vi "ReadDB.vi"() -> ()   [LabVIEW 2018]
uses:
  <vilib>/addons/database/Connection.llb/DB Tools Open Connec (Path).vi
  <vilib>/addons/database/_DB Variant To Data/Database Variant To Data.xnode
  <vilib>/addons/database/NI_Database_API.lvlib
panel:
  out "条目数":i32
  out "data":T1(array[cluster])
  out "error out":errorcluster
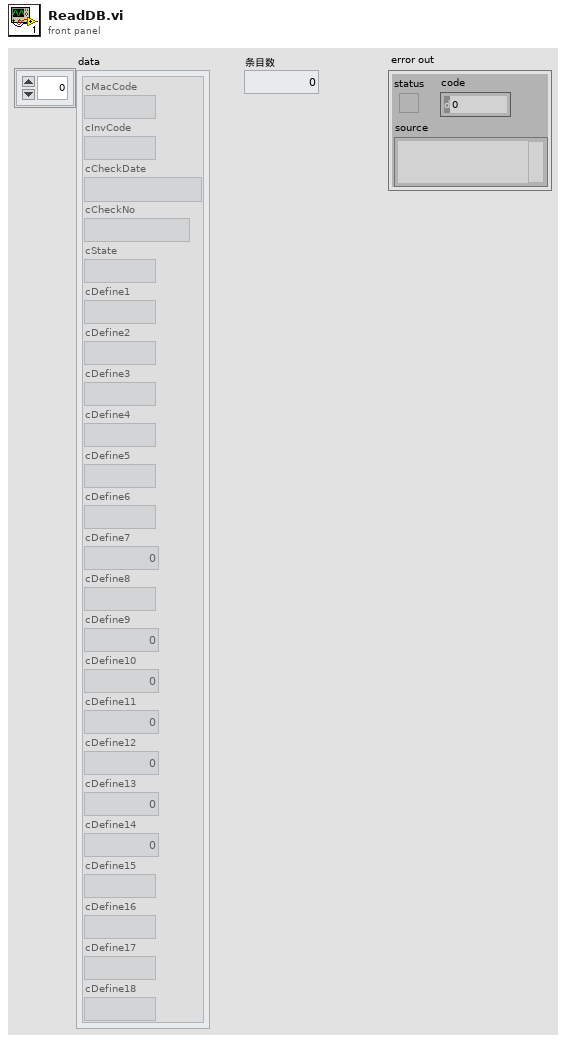
[diagram p1: front panel]
types:
  T1 = cluster{"cMacCode":string, "cInvCode":string, "cCheckDate":string, "cCheckNo":string, "cState":string, "cDefine1":string, "cDefine2":string, "cDefine3":string, "cDefine4":string, "cDefine5":string, "cDefine6":string, "cDefine7":dbl, "cDefine8":string, "cDefine9":dbl, "cDefine10":dbl, "cDefine11":dbl, "cDefine12":dbl, "cDefine13":dbl, "cDefine14":dbl, "cDefine15":string, "cDefine16":string, "cDefine17":string, "cDefine18":string}[]
  T2 = typedef "NI_Database_API.lvlib/Conn ObjectReference.ctl" = refnum<k1>
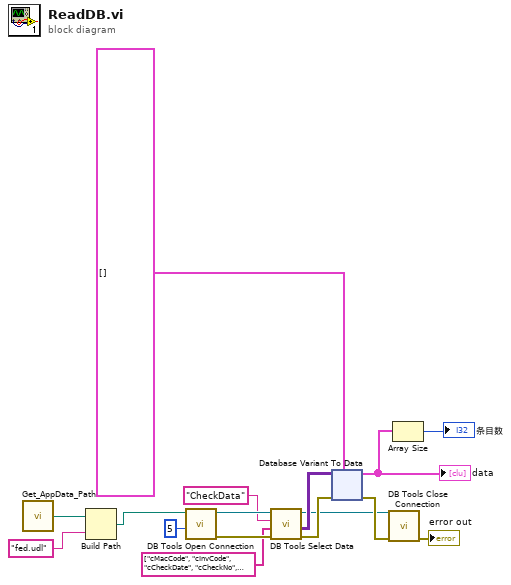
[diagram p0: block diagram]
diagram:
  n1 = call "Get_AppData_Path.vi"() -> ("path"=w15:path)  [unwired: 1 in]
  n2 = Build Path(base path=w15, name or relative path="fed.udl" ("名称或相对路径")) -> (appended path=w14:path)
  n3 = call-poly <vilib>:"DB Tools Open Connection.vi"("connection timeout (15)"=5, "connection information"=w14) -> ("error out"=w10:errorcluster, "connection reference"=w11:T2)  [unwired: 6 in]
  n4 = call <vilib>:"DB Tools Select Data.vi"("error in (no error)"=w10, "columns"=string[] ["cMacCode", "cInvCode", "cCheckDate", "cCheckNo", "cState", "cDefine1", "cDefine2", "cDefine3", "cDefine4", "cDefine5", "cDefine6", "cDefine7", "cDefine8", "cDefine9", "cDefine10", "cDefine11", "cDefine12", "cDefine13", "cDefine14", "cDefine15", "cDefine16", "cDefine17", "cDefine18"] ("Columns"), "table"="CheckData", "connection reference"=w11) -> ("error out"=w8:errorcluster, "data"=w6:variant[][], "connection reference out"=w5:T2)  [unwired: 2 in]
  n5 = xnode "Database Variant To Data"("database variant"=w6, "error in (no error)"=w8, "type"=T1 []) -> ("data"=w2:T1, "error out"=w7:errorcluster)
  "data" <- w2
  n6 = call <vilib>:"DB Tools Close Connection.vi"("error in (no error)"=w7, "connection reference"=w5) -> ("error out"=→"error out":errorcluster)  [unwired: 5 in]
  n7 = Array Size(array=w2) -> (size(s)=→"条目数":i32)
